vi "CreateDefaultLibraryBanner.vi"() -> (3 "Icon":refnum<class "Icon.lvclass">)   [LabVIEW 2014, in "ClassIconTools.lvlib"]
uses:
  ClassIconTools.lvlib
  <vilib>/LabVIEW Icon API/lv_icon/Classes/Icon/Icon.lvclass
  <vilib>/LabVIEW Icon API/API_Rectangle Colors.ctl
  <vilib>/LabVIEW Icon API/LabVIEW Icon API.lvlib
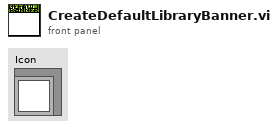
[diagram p1: front panel]
types:
  T1 = cluster{"Size":u8, "Capitalize text":bool, "TextColor":u32}
  T2 = typedef "LabVIEW Icon API.lvlib/API_Rectangle Colors.ctl" = cluster{"Border":u32, "Background":u32}
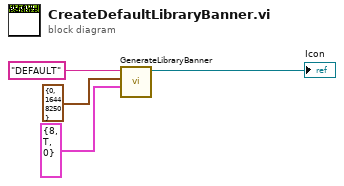
[diagram p0: block diagram]
diagram:
  n1 = call "GenerateLibraryBanner.vi"("Text settings"=T1 {"Size"=8, "Capitalize text"=TRUE, "TextColor"=0}, "Rectangle colors (black, white)"=T2 {"Border"=0, "Background"=16448250}, "Text"="DEFAULT") -> ("Icon.lvlclass out"=→"Icon":refnum<class "Icon.lvclass">)  [unwired: 6 in, 2 out]
